vi "GetPressureSensors.vi"(8 "error in (no error)":errorcluster, 10 "Settings in":T2, 11 "refnum":T1) -> (0 "error out":errorcluster, 2 "Settings out":T2, 3 "refnum out":T1)   [LabVIEW 2026]
uses:
  Settings.ctl
  Acquisition/Hardware Configuration.ctl
  Logging/Logging Configuration.ctl
  <vilib>/Utility/config.llb/Config Data RefNum.ctl
  <vilib>/Utility/config.llb/Read Key (String).vi
  <vilib>/Utility/config.llb/NI_LVConfig.lvlib
  Acquisition/Acquisition.lvlib
  Logging/Logging.lvlib
  Settings.lvlib
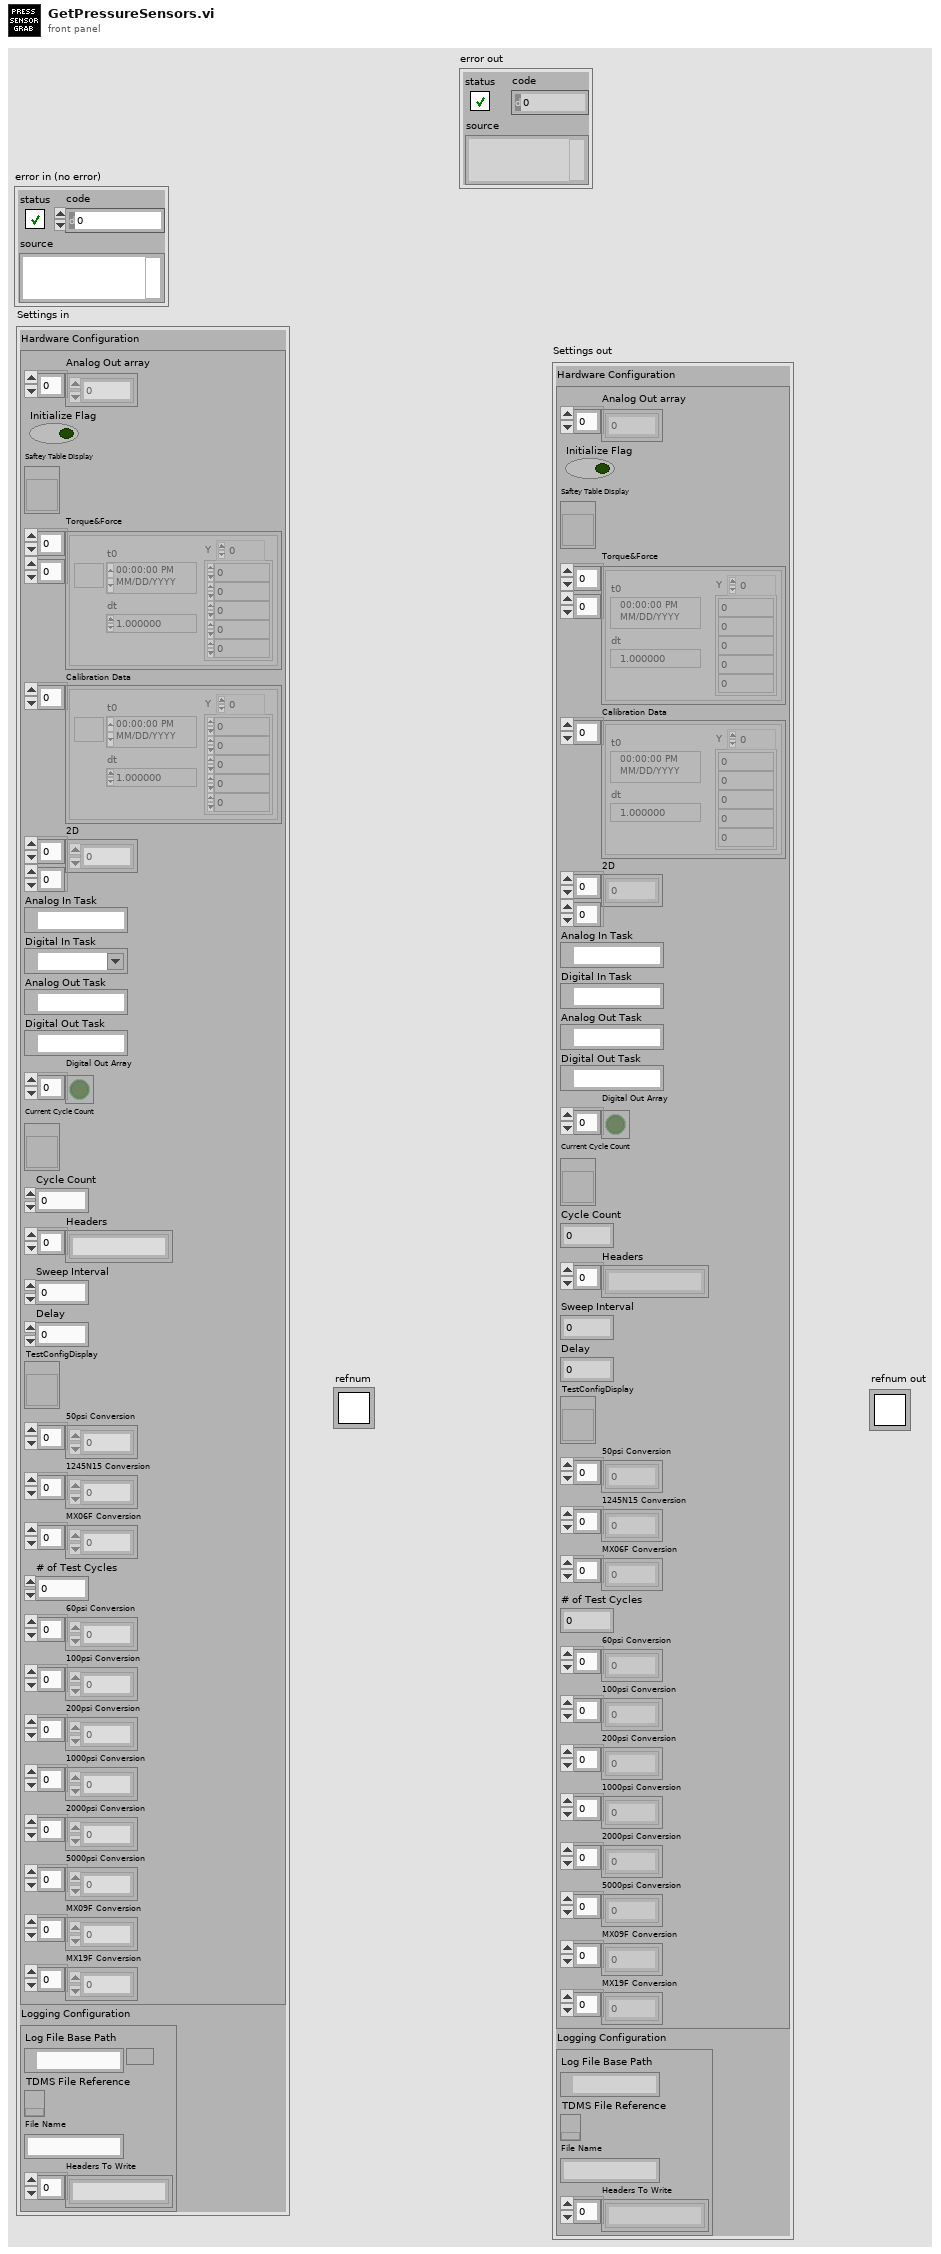
[diagram p1: front panel]
types:
  T1 = typedef "NI_LVConfig.lvlib/Config Data RefNum.ctl" = refnum<k1>
  T2 = typedef "Settings.lvlib/Settings.ctl" = cluster{"Hardware Configuration":T3, "Logging Configuration":T4}
  T3 = typedef "Acquisition.lvlib/Hardware Configuration.ctl" = cluster{"Analog Out array":dbl[], "Initialize Flag":bool, "Saftey Table Display":refnum<vi>, "Torque&Force":waveform(dbl)[][], "Calibration Data":waveform(dbl)[], "2D":dbl[][], "Analog In Task":refnum<k21>, "Digital In Task":refnum<k21>, "Analog Out Task":refnum<k21>, "Digital Out Task":refnum<k21>, "Digital Out Array":bool[], "Current Cycle Count":refnum<vi>, "Cycle Count":u64, "Headers":string[], "Sweep Interval":u64, "Delay":u64, "TestConfigDisplay":refnum<vi>, "50psi Conversion":dbl[], "1245N15 Conversion":dbl[], "MX06F Conversion":dbl[], "# of Test Cycles":u64, "60psi Conversion":dbl[], "100psi Conversion":dbl[], "200psi Conversion":dbl[], "1000psi Conversion":dbl[], "2000psi Conversion":dbl[], "5000psi Conversion":dbl[], "MX09F Conversion":dbl[], "MX19F Conversion":dbl[]}
  T4 = typedef "Logging.lvlib/Logging Configuration.ctl" = cluster{"Log File Base Path":path, "TDMS File Reference":refnum<k34>, "File Name":string, "Headers To Write":string[]}
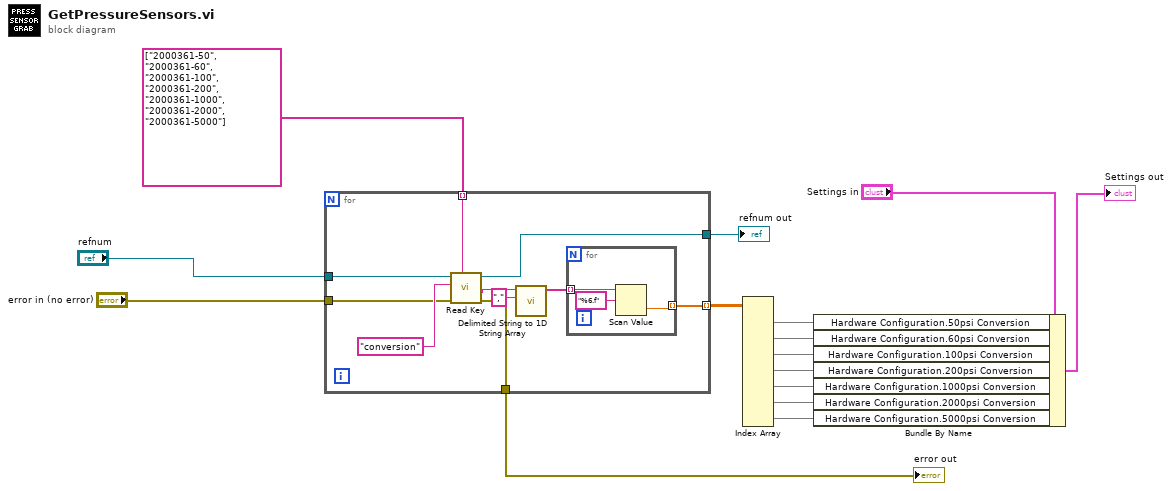
[diagram p0: block diagram]
diagram:
  n1 = for {
    tunnel: string[] ["2000361-50", "2000361-60", "2000361-100", "2000361-200", "2000361-1000", "2000361-2000", "2000361-5000"] ("section") -> [w25] mode=indexing
    tunnel: "error in (no error)" -> [w23]
    tunnel: "refnum" -> [w22]
    tunnel: [w18] -> w12 mode=indexing
    tunnel: [w17] -> w2
    tunnel: [w16] -> w1
    n2 = call-poly <vilib>:"Read Key.vi"("section"=w25, "error in (no error)"=w23, "key"="conversion", "refnum"=w22) -> ("error out"=w16:errorcluster, "value"=w19:string, "refnum out"=w17:T1)  [unwired: 4 in, 1 out]
    n3 = call <vilib>:"Delimited String to 1D String Array.vi"("delimiter"=",", "delimited string"=w19) -> ("string array"=w20:string[])  [unwired: 9 in]
    n4 = for {
      tunnel: w20 -> [w28] mode=indexing
      tunnel: [w26] -> w18 mode=indexing
      n5 = Scan Value(string=w28, format string="%6.f") -> (value=w26:dbl)  [unwired: 1 in, 1 out]
    }
  }
  "refnum out" <- w2
  "error out" <- w1
  n6 = Index Array(array=w12) -> (element #1=w11:dbl[], element #2=w10:dbl[], element #3=w9:dbl[], element #4=w8:dbl[], element #5=w7:dbl[], element #6=w6:dbl[], element #7=w5:dbl[])  [unwired: 14 in]
  n7 = Bundle By Name(cluster="Settings in", "Hardware Configuration.50psi Conversion"=w11, "Hardware Configuration.60psi Conversion"=w10, "Hardware Configuration.100psi Conversion"=w9, "Hardware Configuration.200psi Conversion"=w8, "Hardware Configuration.1000psi Conversion"=w7, "Hardware Configuration.2000psi Conversion"=w6, "Hardware Configuration.5000psi Conversion"=w5) -> (→"Settings out":T2)
